vi "Read App Ref.vi"(8 "error in (no error)":errorcluster, 11 "FileConverterBase in":refnum<class "FileConverterBase.lvclass">) -> (0 "error out":errorcluster, 2 "App Ref":refnum<vi>, 3 "FileConverterBase out":refnum<class "FileConverterBase.lvclass">)   [LabVIEW 2017, in "FileConverterBase.lvclass"]
uses:
  FileConverterBase.lvclass
  FileConverterBase.lvclass/FileConverterBase.ctl
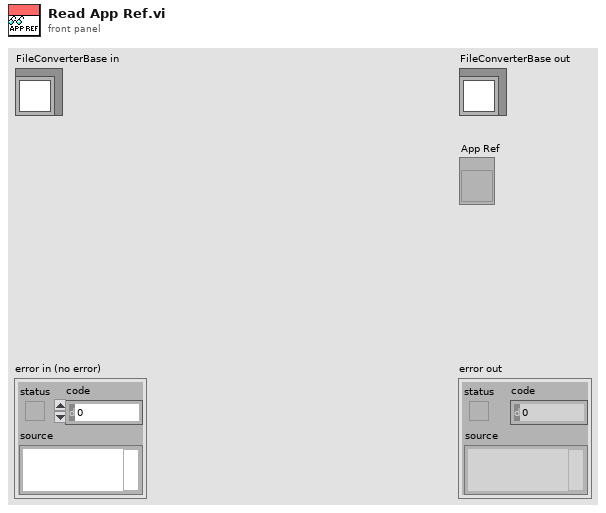
[diagram p1: front panel]
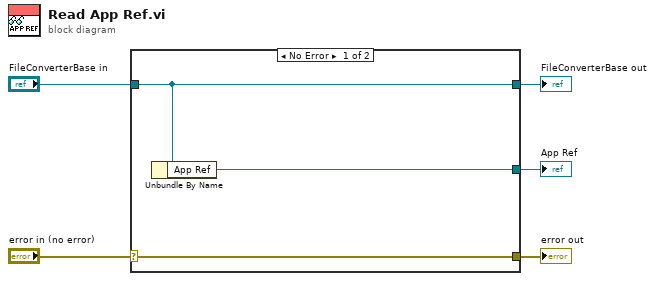
[diagram p0: block diagram]
diagram:
  n1 = case shown="No Error" "error in (no error)" {
    selector: "error in (no error)" -> [w8 w9]
    tunnel: [w8 w9] -> w4
    tunnel: [w7 w10] -> w2
    tunnel: "FileConverterBase in" -> [w7 w10]
    tunnel: [w6 _] -> w1
    frame No Error {
      n2 = Unbundle By Name(w7) -> ("App Ref"=w6:refnum<vi>)
    }
    frame Error {
    }
  }
  "error out" <- w4
  "FileConverterBase out" <- w2
  "App Ref" <- w1
